vi "Reserve.vi"() -> (1 "Don't move motors while reserved":dbl, 2 "Numeric":dbl, 3 "ignore previous (F)":bool)   [LabVIEW 2015]
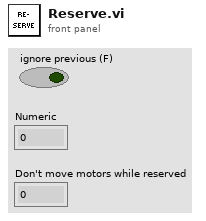
[diagram p1: front panel]
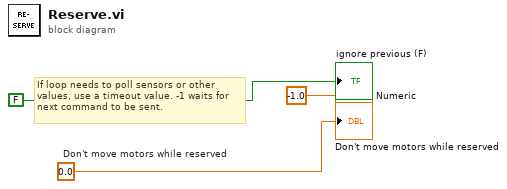
[diagram p0: block diagram]
diagram:
  w3 = 0.0  # Don't move motors while reserved
  # "If loop needs to poll sensors or other\nvalues, use a timeout value. -1 waits for\nnext command to be sent."
  "Don't move motors while reserved" <- w3
  "ignore previous (F)" <- FALSE ("ignore previous (F)")
  "Numeric" <- -1.0
